vi "Temp_SUBVI.vi"() -> (11 "27\n27":bool)   [LabVIEW 2022 SP3]
panel:
  out "28":bool
  out "29":bool
  out "30":bool
  out "Waveform Chart":dbl(graph)
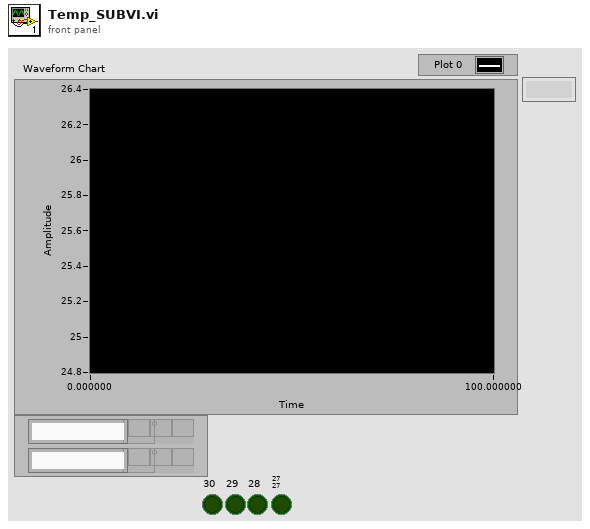
[diagram p1: front panel]
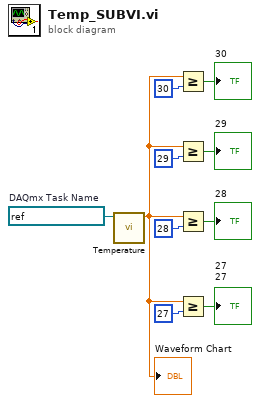
[diagram p0: block diagram]
diagram:
  w2 = refnum<k21> "Temp Sensor"  # DAQmx Task Name
  n1 = call "Temperature.vi"("Refnum in"=w2) -> ("data"=w1:dbl)  [unwired: 10 in]
  "Waveform Chart" <- w1
  n2 = Greater Or Equal?(x=w1, y=30) -> (x >= y?=→"30":bool)
  n3 = Greater Or Equal?(x=w1, y=29) -> (x >= y?=→"29":bool)
  n4 = Greater Or Equal?(x=w1, y=28) -> (x >= y?=→"28":bool)
  n5 = Greater Or Equal?(x=w1, y=27) -> (x >= y?=→"27\n27":bool)
